vi "Value Options Calc.vi"(10 "Options":T1, 11 "Value":string) -> (3 "Value":string)   [LabVIEW 2020, in "BlueVariantView.lvlib"]
uses:
  BlueVariantView.lvlib
  API/Typedefs/Options.ctl
  API/Typedefs/ValueOptions.ctl
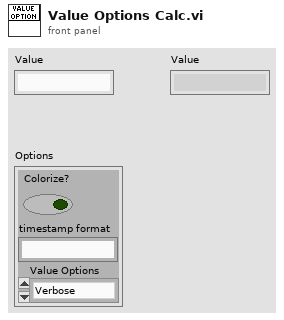
[diagram p1: front panel]
types:
  T1 = typedef "BlueVariantView.lvlib/Options.ctl" = cluster{"Colorize?":bool, "timestamp format":string, "Value Options":T2}
  T2 = typedef "BlueVariantView.lvlib/ValueOptions.ctl" = enum16{"Verbose", "Data only"}
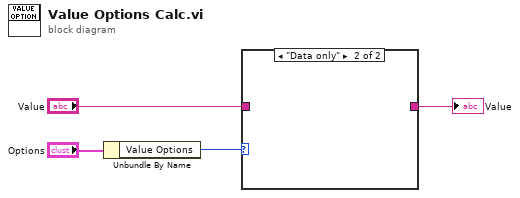
[diagram p0: block diagram]
diagram:
  n1 = Unbundle By Name("Options") -> ("Value Options"=w3:T2)
  n2 = case shown="\"Data only\"" w3 {
    tunnel: [w5 _] -> w2
    tunnel: "Value" -> [w5 _]
    frame "Verbose" {
    }
    frame "Data only" {
    }
  }
  "Value" <- w2
